vi "transmitUDP.vi"(8 "error in (no error)":errorcluster, 10 "data in":string, 11 "UDP Network Connection in":refnum<k16>) -> (0 "error out":errorcluster, 3 "UDP Network Connection out":refnum<k16>)   [LabVIEW 2017, in "communicateMLC.lvlib"]
doc: "This VI sends data to the PC via UDP. The PC IP is set to 172.22.11.1 and the PC listening port is 65530"
uses:
  communicateMLC.lvlib
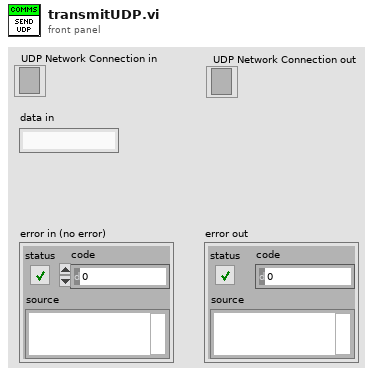
[diagram p1: front panel]
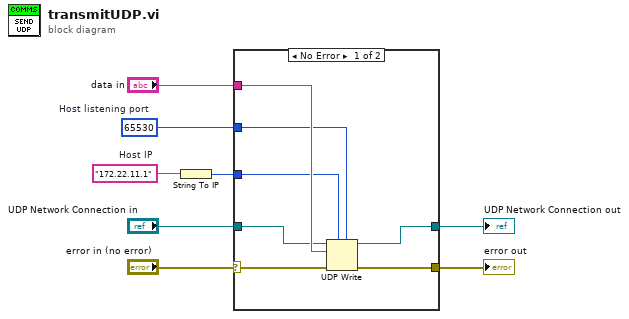
[diagram p0: block diagram]
diagram:
  w3 = u16 65530  # Host listening port
  w4 = "172.22.11.1"  # Host IP
  n1 = String To IP(1:w4) -> (0:w2:u32)
  n2 = case shown="No Error" "error in (no error)" {
    selector: "error in (no error)" -> [w9 w17]
    tunnel: "data in" -> [w15 _]
    tunnel: [w14 w17] -> w7
    tunnel: [w13 w16] -> w6
    tunnel: "UDP Network Connection in" -> [w12 w16]
    tunnel: w3 -> [w11 _]
    tunnel: w2 -> [w10 _]
    frame No Error {
      n3 = UDP Write(address=w10, port or service name=w11, connection ID=w12, data in=w15, 8:w9) -> (error out=w14:errorcluster, 3:w13:refnum<k16>)  [unwired: 1 in]
    }
    frame Error {
    }
  }
  "error out" <- w7
  "UDP Network Connection out" <- w6
